vi "Destroy And Stop Process.vi"(8 "error in (no error)":errorcluster, 11 "Interlock Q Class in":refnum<class "Interlock Q Class.lvclass">) -> (0 "error out":errorcluster, 3 "Interlock Q Class out":refnum<class "Interlock Q Class.lvclass">)   [LabVIEW 2022 SP3, in "Interlock Q Class.lvclass"]
uses:
  Interlock Q Class.lvclass
  Interlock Q Class.lvclass/Interlock Q Class.ctl
  <vilib>/ActorFramework/Message Enqueuer/Message Enqueuer.lvclass/Message Enqueuer.ctl
  <vilib>/ActorFramework/Message Enqueuer/Enqueue.vi
  <vilib>/ActorFramework/Stop Msg/Stop Msg.lvclass
  C:/Program Files/National Instruments/LabVIEW 2022/vi.lib/ActorFramework/Message/Message.lvclass
  <vilib>/ActorFramework/Message Priority Queue/Priority Enqueue.vi
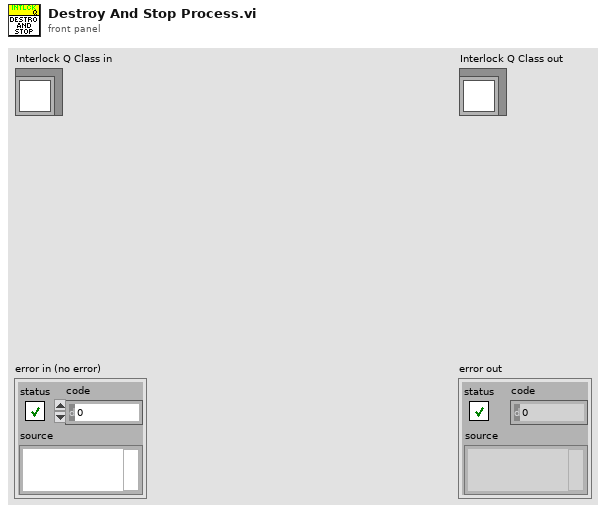
[diagram p1: front panel]
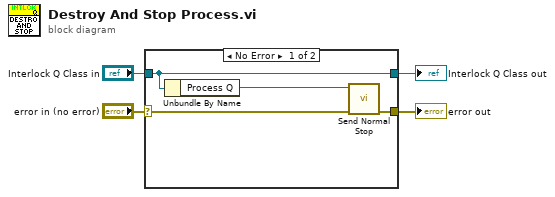
[diagram p0: block diagram]
diagram:
  n1 = case shown="No Error" "error in (no error)" {
    selector: "error in (no error)" -> [w6 w10]
    tunnel: [w5 w10] -> w3
    tunnel: [w8 w9] -> w1
    tunnel: "Interlock Q Class in" -> [w8 w9]
    frame No Error {
      n2 = Unbundle By Name(w8) -> ("Process Q"=w7:refnum<class "Message Enqueuer.lvclass">)
      n3 = call <vilib>:"Send Normal Stop.vi"("error in (no error)"=w6, "Message Enqueuer"=w7) -> ("error out"=w5:errorcluster)  [unwired: 9 in]
    }
    frame Error {
    }
  }
  "error out" <- w3
  "Interlock Q Class out" <- w1
